vi "CSUWebClient.vi"(4 "Scan Period":dbl format="%.2f", 5 "Previous Scan Value":dbl format="%.2f", 6 "Present scan array":dbl[](array[numeric]) format="%.2f", 7 "Value to Output":dbl format="%.2f", 8 "Ch Description":T1={"Ch Name"="", "Type"="", "Function"=enum."Analogue Input", "Ch State"=enum."On", "Calibration type"=enum."Raw", "A"=0.0, "B"=0.0, "C"=0.0, "D"=0.0, "Comments"="", "Address"={"Main"=0, "Ch."=0, "Sub"=0, "Port Name"=""}, "String"="", "Duty"=65535} {"Duty" format="%.0b"; "D" format="%#_5g"; "C" format="%#_5g"; "B" format="%#_5g"; "A" format="%#_5g"}, 9 "Ch names":string[](array[string])) -> (0 "Scan comment":string, 1 "Output":dbl format="%.3f")   [LabVIEW 2011]
uses:
  ADAM Client/Sub VIs/ADAM Controls/Ch_description_ADAM.ctl
  ADAM Client/Sub VIs/ADAM Controls/Module_type_ADAM.ctl
  ADAM Client/Sub VIs/ADAM Controls/Function_ADAM.ctl
  ADAM Client/Sub VIs/ADAM Controls/Channel_State.ctl
  ADAM Client/Sub VIs/ADAM Controls/Calib_type_ADAM.ctl
  ADAM Client/Sub VIs/ADAM Controls/Address.ctl
  ADAM Client/Sub VIs/ADAM Controls/Remember_value_mode.ctl
panel:
  out "Time Of Value (s)":dbl format="%.2f"
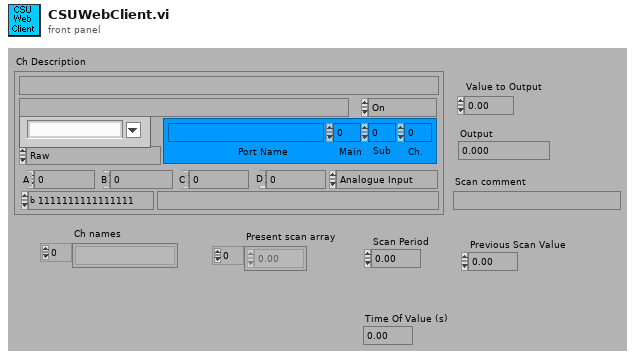
[diagram p1: front panel]
types:
  T1 = typedef "Ch_description_ADAM.ctl" = cluster{"Ch Name":string, "Type":T2, "Function":T3, "Ch State":T4, "Calibration type":T5, "A":dbl, "B":dbl, "C":dbl, "D":dbl, "Comments":string, "Address":T6, "String":string, "Duty":u16}
  T2 = typedef "Module_type_ADAM.ctl" = string
  T3 = typedef "Function_ADAM.ctl" = enum16{"Analogue Input", "Digital Input", "Event counter", "Event rate", "Analogue Output", "Digital Output", "Relay Output"}
  T4 = typedef "Channel_State.ctl" = enum16{"On", "Off", "Always On", "Always Off"}
  T5 = typedef "Calib_type_ADAM.ctl" = enum16{"Raw", "Bx + A", "Cx^2 + Bx + A", "Dx^3 + Cx^2 + Bx + A", "In Band", "Hi-Tec Q", "Hi-Tec M_dot", "Text"}
  T6 = typedef "Address.ctl" = cluster{"Main":i32, "Ch.":i32, "Sub":i32, "Port Name":string}
  T7 = typedef "Remember_value_mode.ctl" = enum16{"Read only", "Read and Write"}
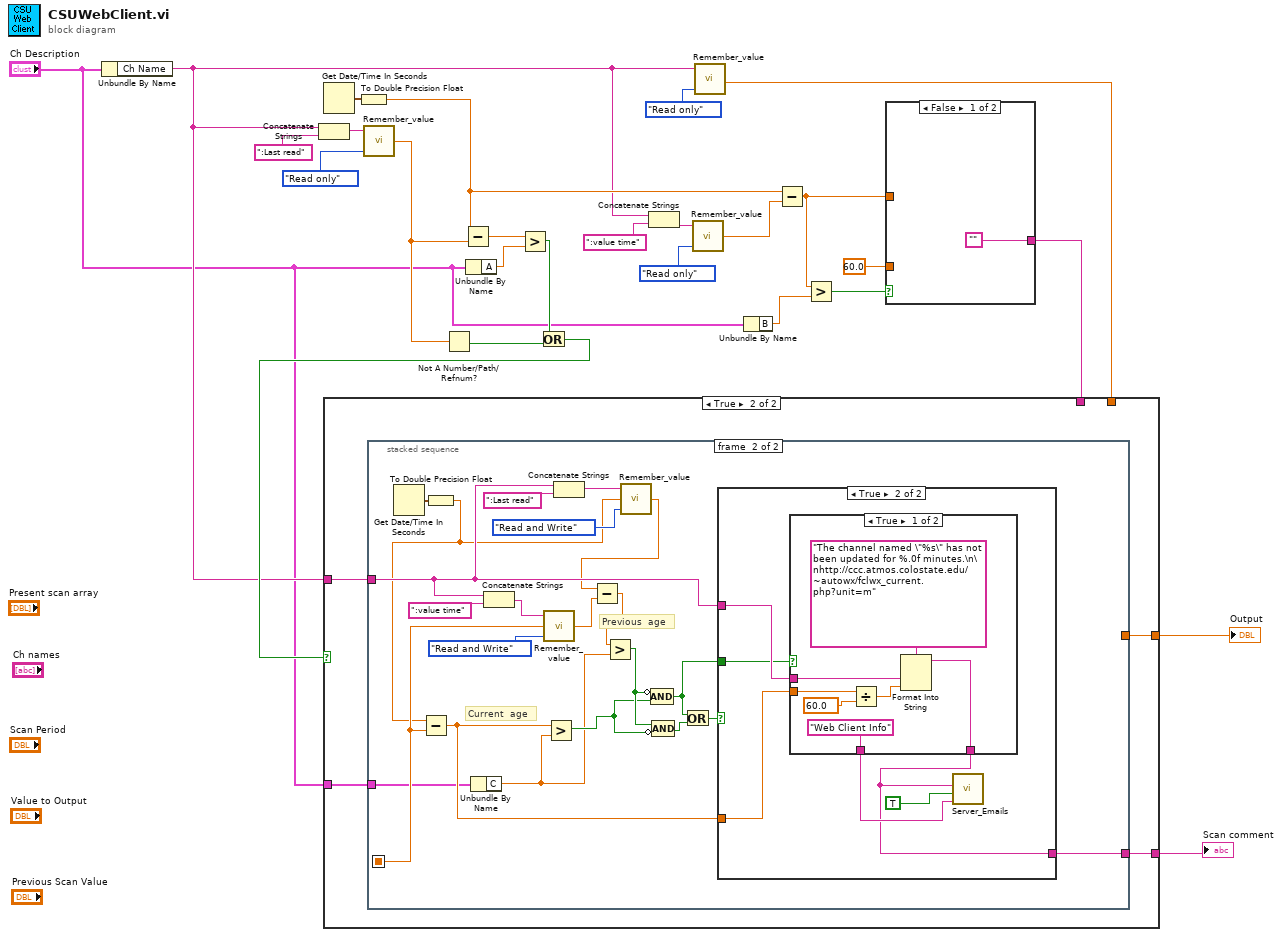
[diagram p0: block diagram]
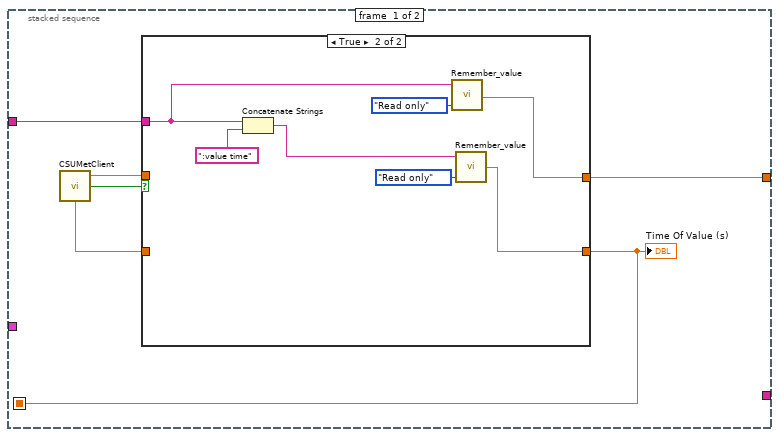
[diagram p3: hidden frame]
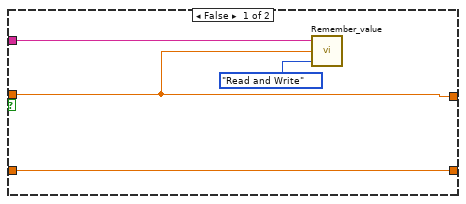
[diagram p4: hidden frame]
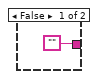
[diagram p5: hidden frame]
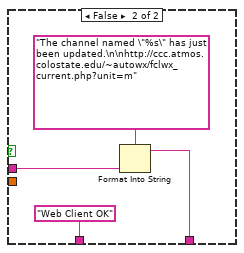
[diagram p6: hidden frame]
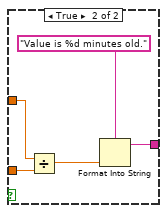
[diagram p7: hidden frame]
diagram:
  n1 = Unbundle By Name("Ch Description") -> ("Ch Name"=w8:string)
  n2 = Concatenate Strings(w8, ":Last read" ("Substring")) -> (w23:string)
  n3 = Get Date/Time In Seconds() -> (seconds since 1Jan1904=w17:timestamp)
  n4 = To Double Precision Float(number=w17) -> (double precision float=w15:dbl)
  n5 = call "Remember_value.vi"("Mode"=Remember_value_mode."Read only", "Ch name"=w23) -> ("Output Value"=w22:dbl)  [unwired: 1 in]
  n6 = Not A Number/Path/Refnum?(number/path/refnum=w22) -> (NaN/Path/Refnum?=w20:bool)
  n7 = Subtract(x=w15, y=w22) -> (x-y=w26:dbl)
  n8 = Unbundle By Name("Ch Description") -> ("A"=w3:dbl)
  n9 = Greater?(x=w26, y=w3) -> (0:w21:bool)
  n10 = Or(x=w21, y=w20) -> (x .or. y?=w9:bool)
  n11 = Concatenate Strings(w8, ":value time" ("Substring")) -> (w11:string)
  n12 = call "Remember_value.vi"("Mode"=Remember_value_mode."Read only", "Ch name"=w11) -> ("Output Value"=w16:dbl)  [unwired: 1 in]
  n13 = call "Remember_value.vi"("Mode"=Remember_value_mode."Read only", "Ch name"=w8) -> ("Output Value"=w4:dbl)  [unwired: 1 in]
  n14 = Unbundle By Name("Ch Description") -> ("B"=w2:dbl)
  n15 = Subtract(x=w15, y=w16) -> (x-y=w14:dbl)
  n16 = Greater?(x=w14, y=w2) -> (0:w19:bool)
  n17 = case shown="False" w19 {
    tunnel: w14 -> [_ w32]
    tunnel: 60.0 ("y") -> [_ w31]
    tunnel: ["" w29] -> w6
    frame False {
    }
    frame True {
      n18 = Divide(x=w32, y=w31) -> (x/y=w28:dbl)
      n19 = Format Into String(format string="Value is %d minutes old." ("Format String"), w28) -> (resulting string=w29:string)  [unwired: 2 in, 1 out]
    }
  }
  n20 = case shown="True" w9 {
    tunnel: w8 -> [_ w38]
    tunnel: [w34 w37] -> w7
    tunnel: w6 -> [w34 _]
    tunnel: [w33 w36] -> w5
    tunnel: w4 -> [w33 _]
    tunnel: "Ch Description" -> [_ w35]
    frame False {
    }
    frame True {
      n21 = stacked-sequence {
        seq-local: [w44 _] -> [_ w66]
        tunnel: w38 -> [w43 w61]
        tunnel: [_ w58] -> w37
        tunnel: [w39 _] -> w36
        tunnel: w35 -> [_ w56]
        frame #0 {
          n22 = call "CSUMetClient.vi"() -> ("Time Of Value (s)"=w40:dbl, "Error"=w42:bool, "RawPressure/mBar"=w41:dbl)
          n23 = case shown="True" w42 {
            tunnel: [w45 w49] -> w39
            tunnel: [w48 w50] -> w44
            tunnel: w43 -> [w46 w52]
            tunnel: w41 -> [w45 _]
            tunnel: w40 -> [w48 _]
            frame False {
              n24 = call "Remember_value.vi"("Mode"=Remember_value_mode."Read and Write", "Input Value"=w45, "Ch name"=w46) -> ()  [unwired: 1 out]
            }
            frame True {
              n25 = Concatenate Strings(w52, ":value time" ("Substring")) -> (w51:string)
              n26 = call "Remember_value.vi"("Mode"=Remember_value_mode."Read only", "Ch name"=w52) -> ("Output Value"=w49:dbl)  [unwired: 1 in]
              n27 = call "Remember_value.vi"("Mode"=Remember_value_mode."Read only", "Ch name"=w51) -> ("Output Value"=w50:dbl)  [unwired: 1 in]
            }
          }
          "Time Of Value (s)" <- w44
        }
        frame #1 {
          # "Previous  age"
          # "Current  age"
          n28 = Get Date/Time In Seconds() -> (seconds since 1Jan1904=w69:timestamp)
          n29 = To Double Precision Float(number=w69) -> (double precision float=w60:dbl)
          n30 = Subtract(x=w60, y=w66) -> (x-y=w65:dbl)
          n31 = Unbundle By Name(w56) -> ("C"=w57:dbl)
          n32 = Concatenate Strings(w61, ":value time" ("Substring")) -> (w75:string)
          n33 = call "Remember_value.vi"("Mode"=Remember_value_mode."Read and Write", "Input Value"=w66, "Ch name"=w75) -> ("Output Value"=w68:dbl)
          n34 = Greater?(x=w65, y=w57) -> (0:w73:bool)
          n35 = Concatenate Strings(w61, ":Last read" ("Substring")) -> (w62:string)
          n36 = call "Remember_value.vi"("Mode"=Remember_value_mode."Read and Write", "Input Value"=w60, "Ch name"=w62) -> ("Output Value"=w59:dbl)
          n37 = Subtract(x=w59, y=w68) -> (x-y=w67:dbl)
          n38 = Greater?(x=w67, y=w57) -> (0:w74:bool)
          n39 = Compound Arithmetic op=AND(invert w74, w73) -> (w70:bool)
          n40 = Compound Arithmetic op=AND(w74, invert w73) -> (w72:bool)
          n41 = Or(x=w70, y=w72) -> (x .or. y?=w71:bool)
          n42 = case shown="True" w71 {
            tunnel: w65 -> [_ w84]
            tunnel: w61 -> [_ w83]
            tunnel: w70 -> [_ w82]
            tunnel: ["" w79] -> w58
            frame False {
            }
            frame True {
              n43 = case shown="True" w82 {
                tunnel: w84 -> [w89 _]
                tunnel: w83 -> [w91 w95]
                tunnel: [w86 w93] -> w79
                tunnel: ["Web Client Info" ("Subject") "Web Client OK" ("Subject")] -> w80
                frame True {
                  n44 = Divide(x=w89, y=60.0) -> (x/y=w88:dbl)
                  n45 = Format Into String(format string="The channel named \"%s\" has not been updated for %.0f minutes.\n\nhttp://ccc.atmos.colostate.edu/~autowx/fclwx_current.php?unit=m" ("Format String"), w91, w88) -> (resulting string=w86:string)  [unwired: 2 in, 1 out]
                }
                frame False {
                  n46 = Format Into String(format string="The channel named \"%s\" has just been updated.\n\nhttp://ccc.atmos.colostate.edu/~autowx/fclwx_current.php?unit=m" ("Format String"), w95) -> (resulting string=w93:string)  [unwired: 2 in, 1 out]
                }
              }
              n47 = call "Server_Emails.vi"("Message"=w79, "Contact All clients?"=TRUE, "Subject"=w80) -> ()  [unwired: 2 in, 3 out]
            }
          }
        }
      }
    }
  }
  "Scan comment" <- w7
  "Output" <- w5
